vi "UTIL Config Analog Output_Final.vi"(0 "physical channels":tag) -> (1 "sampling info":cluster{"Fs":dbl, "#s":dbl}, 2 "error out":errorcluster, 3 "task out":refnum<k21>)   [LabVIEW 2017]
uses:
  <vilib>/DAQmx/create/channels.llb/DAQmx Create Channel (AO-Voltage-Basic).vi
  <vilib>/DAQmx/configure/timing.llb/DAQmx Timing (Sample Clock).vi
  <resource>/objmgr/daqmx.rc
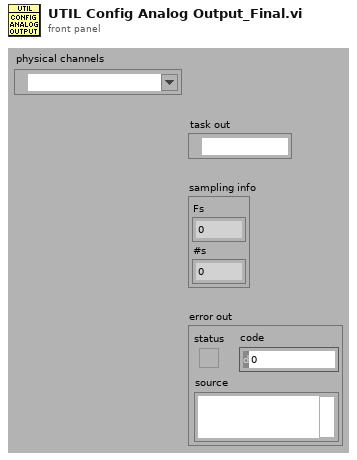
[diagram p1: front panel]
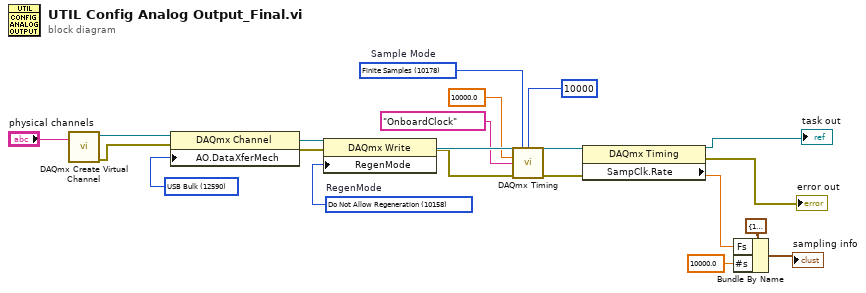
[diagram p0: block diagram]
diagram:
  w2 = 12590 items=["DMA"=10054, "Interrupts"=10204, "Programmed I/O"=10264, "USB Bulk"=12590] ("AO.DataXferMech")
  w12 = 10158 items=["Allow Regeneration"=10097, "Do Not Allow Regeneration"=10158]  # RegenMode
  w10 = 10178 items=["Finite Samples"=10178, "Continuous Samples"=10123, "Hardware Timed Single Point"=12522]  # Sample Mode
  n1 = call-poly <vilib>:"DAQmx Create Virtual Channel.vi"("physical channels"="physical channels") -> ("task out"=w5:refnum<k21>, "error out"=w3:errorcluster)  [unwired: 13 in]
  n2 = property class="DAQmx Channel"(reference=w5, error in=w3, "AO.DataXferMech"=w2) -> (reference out=w9:refnum<k21>, error out=w8:errorcluster)
  n3 = property class="DAQmx Write"(reference=w9, error in=w8, "RegenMode"=w12) -> (reference out=w16:refnum<k21>, error out=w11:errorcluster)
  n4 = call-poly <vilib>:"DAQmx Timing.vi"("task/channels in"=w16, "sample mode"=w10, "samples per channel"=10000, "rate"=10000.0, "source"=tag "OnboardClock" ("Sample Clock Source"), "error in"=w11) -> ("task out"=w14:refnum<k21>, "error out"=w15:errorcluster)  [unwired: 8 in]
  n5 = property class="DAQmx Timing"(reference=w14, error in=w15) -> (reference out=→"task out":refnum<k21>, error out=→"error out":errorcluster, "SampClk.Rate"=w20:dbl)
  n6 = Bundle By Name(cluster=cluster{"Fs":dbl, "#s":dbl} {"Fs"=1000.0, "#s"=1000.0} ("sampling info"), "Fs"=w20, "#s"=10000.0) -> (→"sampling info":cluster{"Fs":dbl, "#s":dbl})
